vi "EX 5-1 Seven Segment Display.vi"() -> ()   [LabVIEW 2011, in "LabVIEW Interface for Arduino.lvlib"]
doc: "An example that uses the digital output pins of the Arduino to control a seven segment display."
uses:
  <vilib>/LabVIEW Interface for Arduino/LabVIEW Interface for Arduino.lvlib
panel:
  in  "Stop":bool
  in  "Time (ms)":u32=500
  in  "String":string="HELLO "
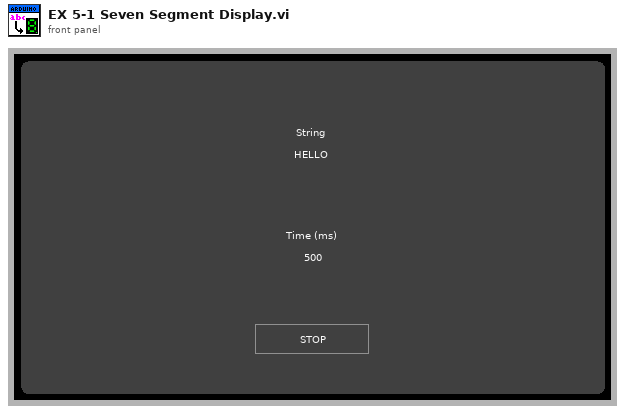
[diagram p1: front panel]
types:
  T1 = typedef "LabVIEW Interface for Arduino.lvlib/Arduino Resource.ctl" = cluster{"VISA resource":refnum<visa-resource-name>, "Board Type":T2, "Connection Type":enum8{"USB / Serial"}, "Bytes Per Packet (15)":u8}
  T2 = typedef "LabVIEW Interface for Arduino.lvlib/Board Type.ctl" = enum16{"Uno", "Dimuelanove w/Atmega 328", "Mega 2560"}
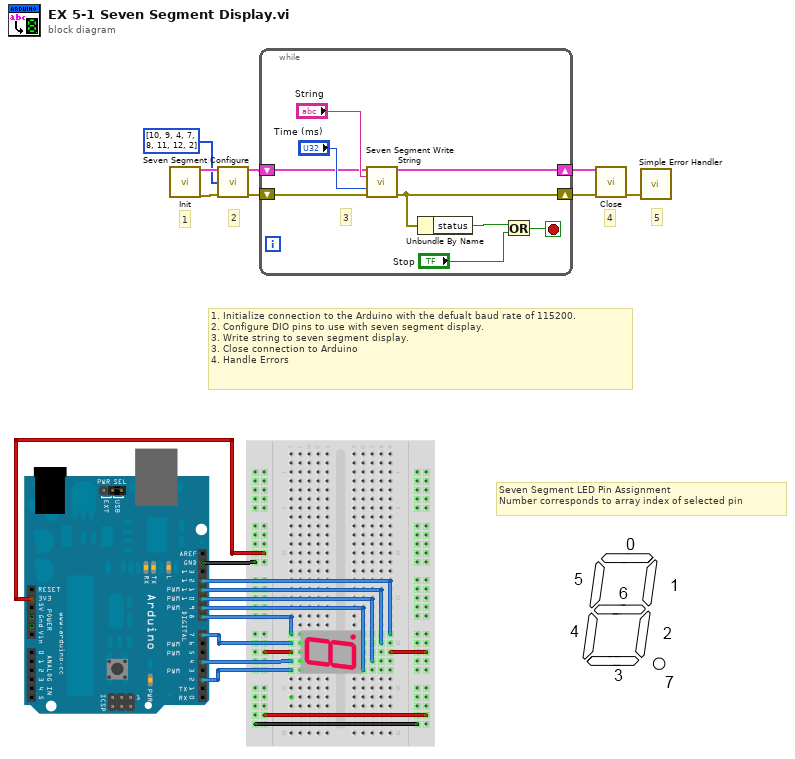
[diagram p0: block diagram]
diagram:
  # "Seven Segment LED Pin Assignment\nNumber corresponds to array index of selected pin"
  # "5"
  # "4"
  # "2"
  # "1"
  # "1. Initialize connection to the Arduino with the defualt baud rate of 115200.\n2. Configure DIO pins to use with seven segment display. \n3. Write string to seven segment display.\n3. Close connection to Arduino\n4. Handle Errors"
  n1 = call <vilib>:"Init.vi"() -> ("Arduino Resource"=w2:T1, "error out"=w5:errorcluster)  [unwired: 18 in]
  n2 = call <vilib>:"Seven Segment Configure.vi"("Arduino Resource"=w2, "Seven Segment Pins"=u8[] [10, 9, 4, 7, 8, 11, 12, 2], "error in"=w5) -> ("Arduino Resource"=w7:T1, "error out"=w6:errorcluster)  [unwired: 11 in]
  n3 = while {
    shift-right: [w17] -> w3
    shift-left: w7 -> [w9]
    shift-right: [w13] -> w8
    shift-left: w6 -> [w16]
    stop <- w12 stop-if-true
    # "3"
    n4 = call <vilib>:"Seven Segment Write String.vi"("Arduino Resource"=w9, "String"="String", "Time ms (500)"="Time (ms)", "error in"=w16) -> ("Arduino Resource"=w17:T1, "error out"=w13:errorcluster)  [unwired: 10 in]
    n5 = Unbundle By Name(w13) -> ("status"=w11:bool)
    n6 = Or(x=w11, y="Stop") -> (x .or. y?=w12:bool)
  }
  n7 = call <vilib>:"Close.vi"("Arduino Resource"=w3, "error in"=w8) -> ("error out"=w4:errorcluster)  [unwired: 13 in]
  n8 = call <vilib>:"Simple Error Handler.vi"("error in (no error)"=w4) -> ()  [unwired: 4 in, 5 out]
